vi "DWSPT5_Read.vi"(8 "错误输入（无错误）":errorcluster, 11 "VISA resource name":refnum<visa-resource-name> caption="VISA资源名称") -> (0 "error out":errorcluster caption="错误输出", 3 "Data":T1)   [LabVIEW 2017]
panel:
  out "长度 2":i32
  out "长度":i32
  out "HumidityValue":string
  out "TemperatureValue":string
  in  "Command":string="010300010002\n"
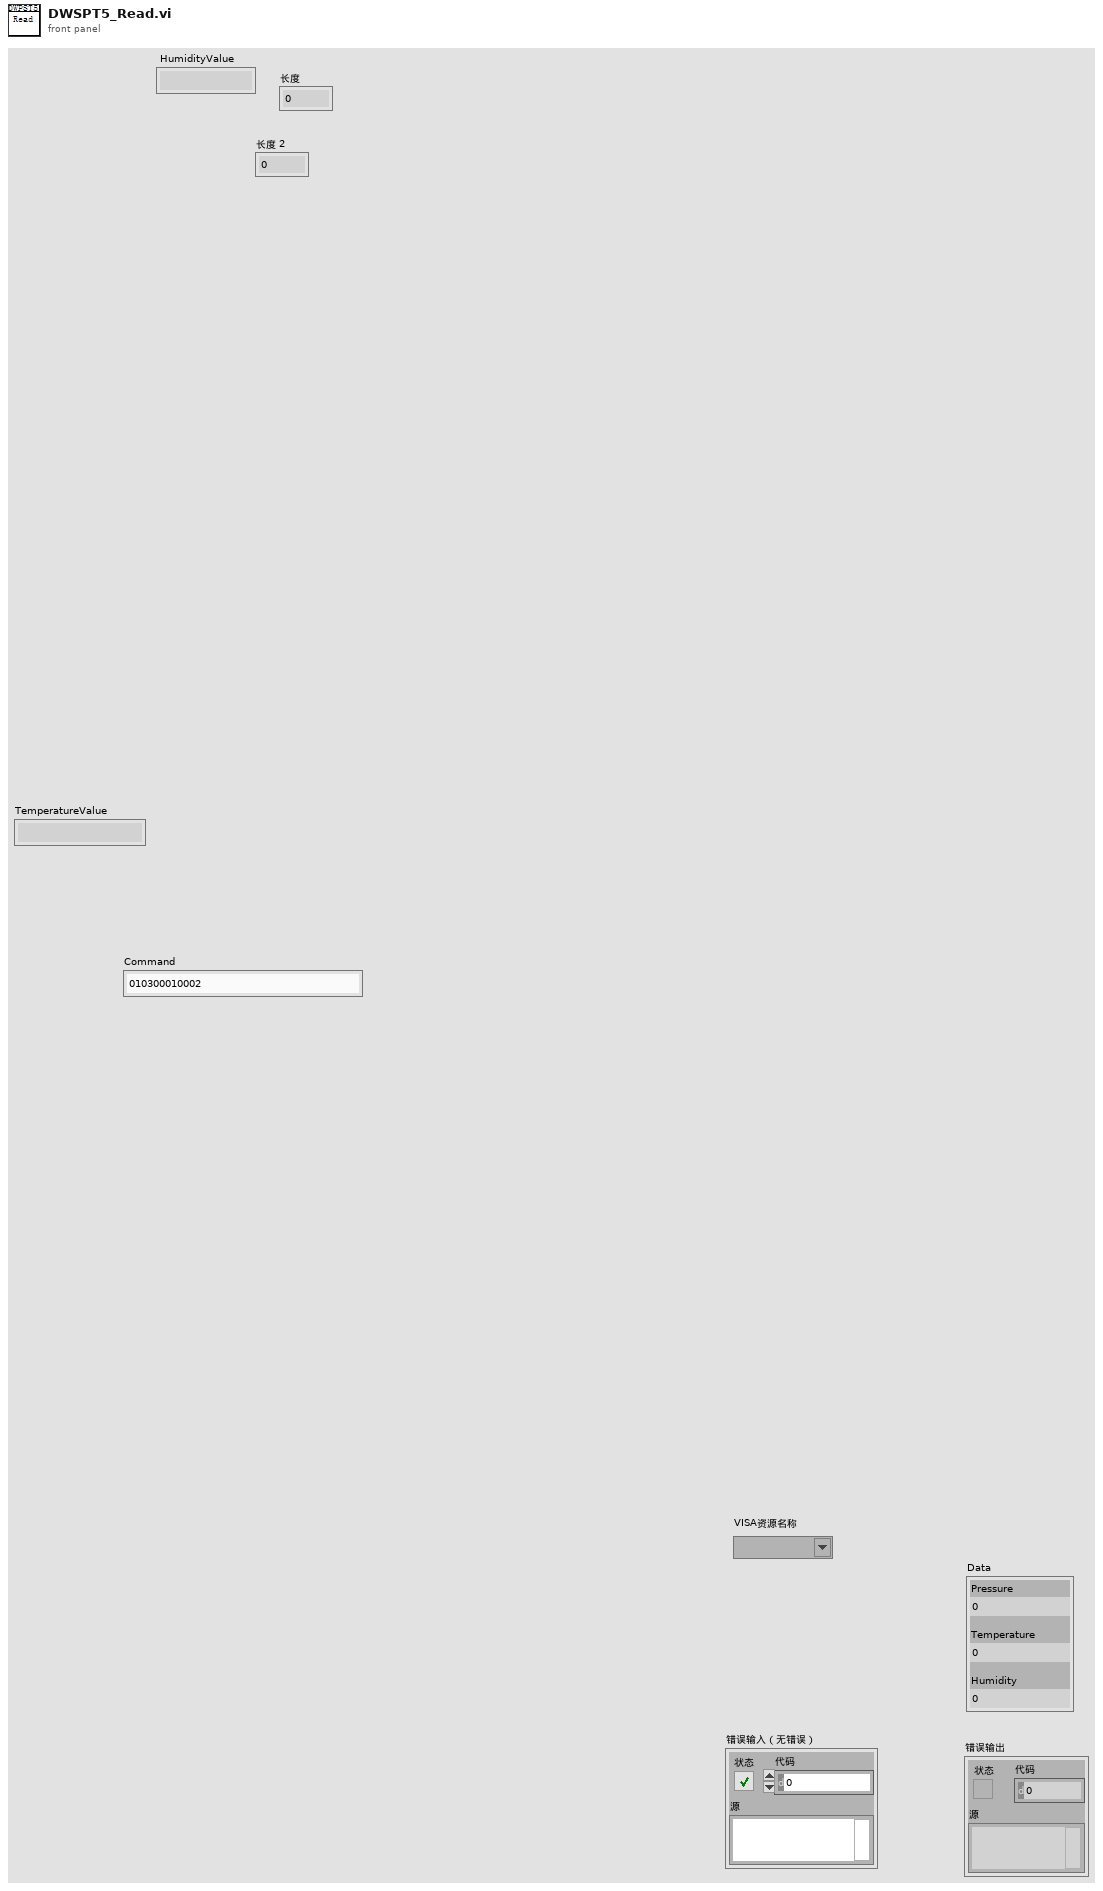
[diagram p1: front panel]
types:
  T1 = cluster{"Pressure":dbl, "Temperature":dbl, "Humidity":dbl}
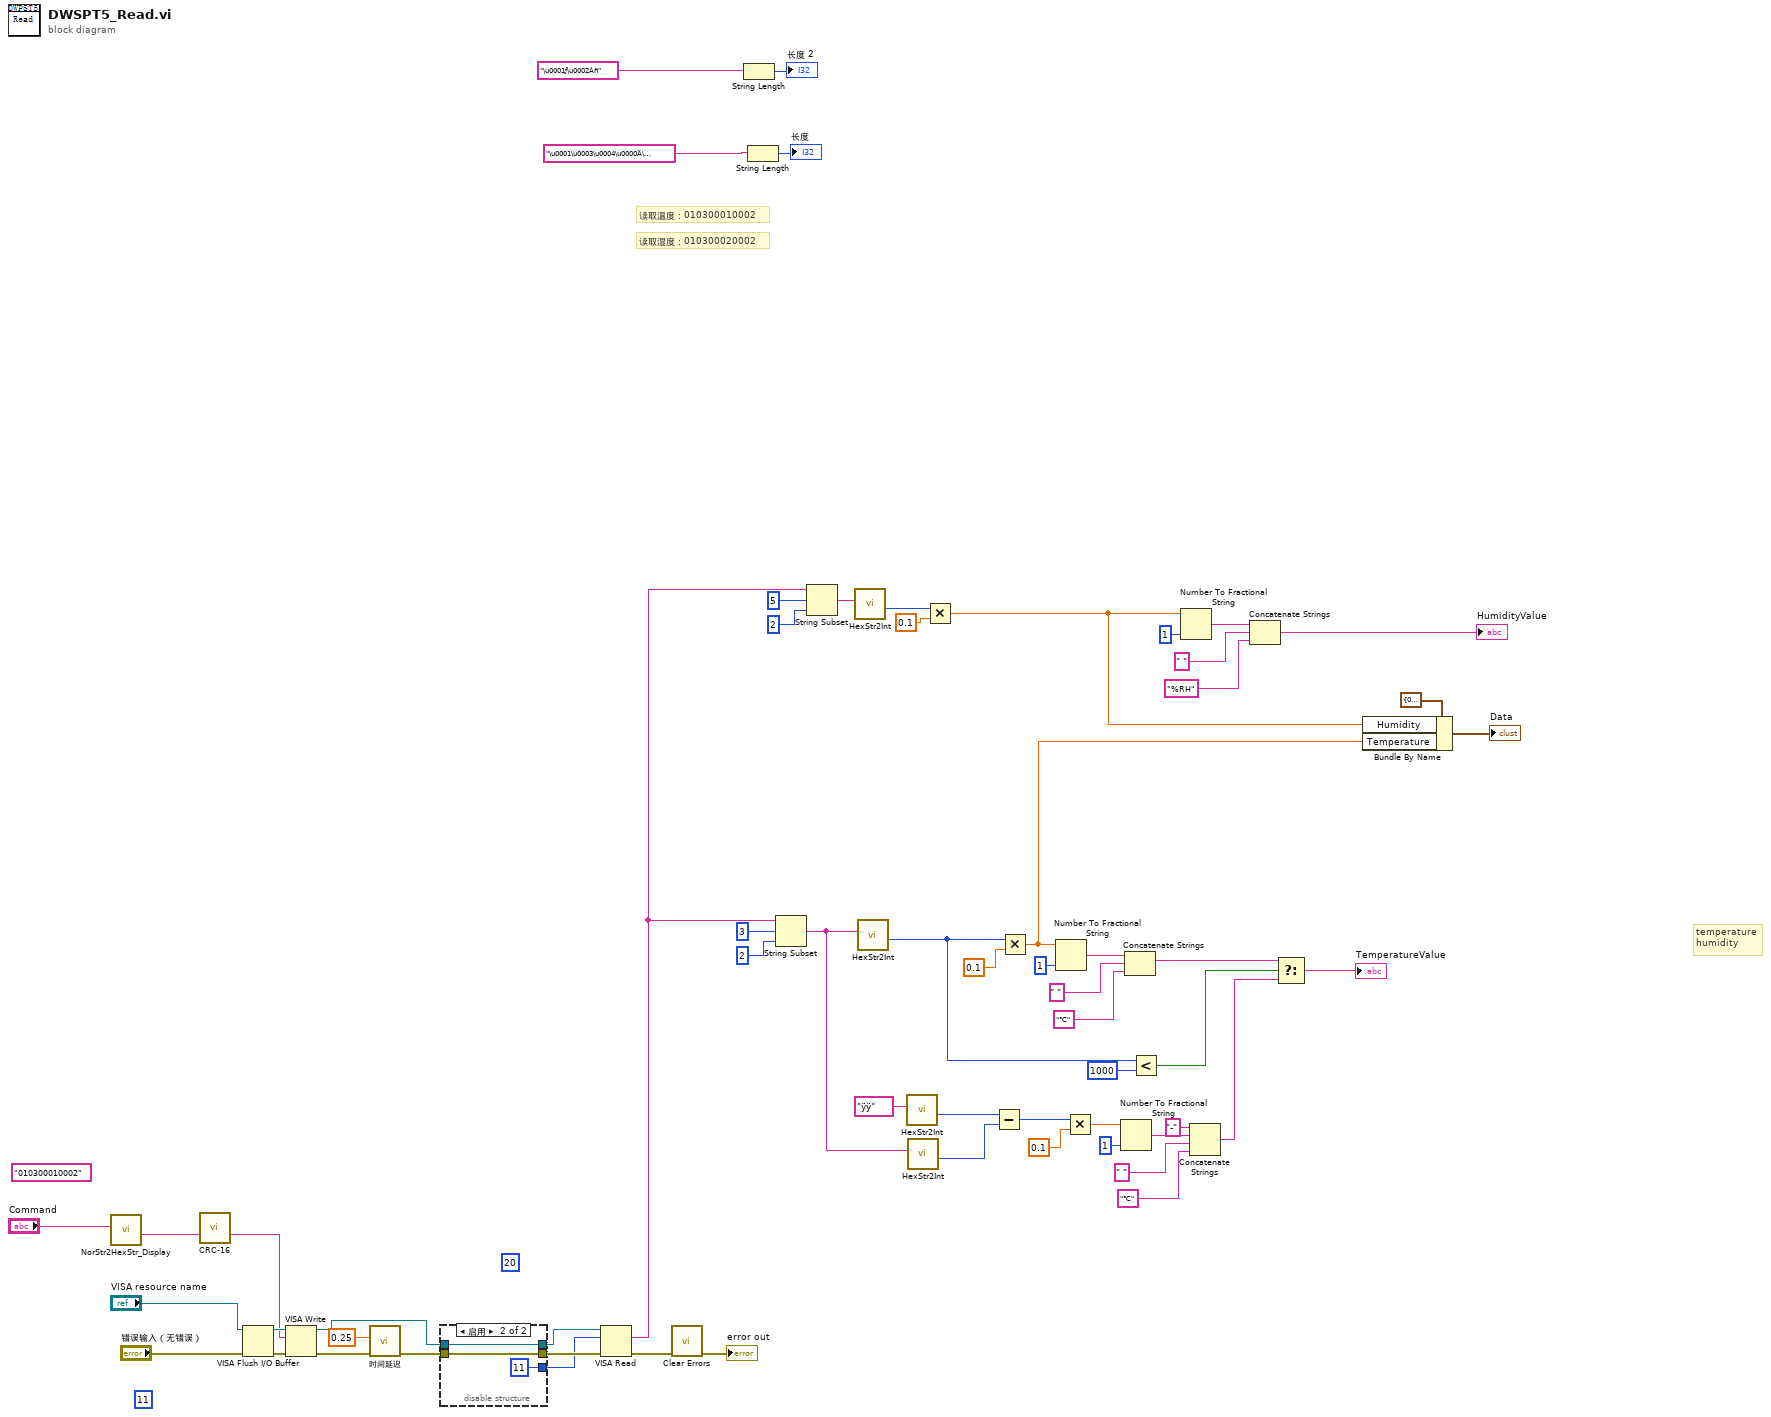
[diagram p0: block diagram]
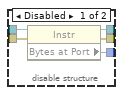
[diagram p2: hidden frame]
diagram:
  (unwired) "010300010002" ("Command 2")
  (unwired) u32 20 ("字节总数")
  (unwired) u32 11 ("byte count")
  # "读取湿度：010300020002"
  # "读取温度：010300010002"
  # "temperature\nhumidity"
  n1 = call "NorStr2HexStr_Display.vi"("Normal Display"="Command") -> ("Hex Display"=w45:string)  [unwired: 10 in]
  n2 = call "CRC-16.vi"("string_hex"=w45) -> ("string&CRC-16"=w44:string)  [unwired: 14 in]
  n3 = VISA Flush I/O Buffer(VISA resource name="VISA resource name", error in (no error)="错误输入（无错误）") -> (VISA resource name out=w60:refnum<visa-resource-name>, error out=w58:errorcluster)  [unwired: 1 in]
  n4 = VISA Write(VISA resource name=w60, write buffer=w44, error in (no error)=w58) -> (VISA resource name out=w50:refnum<visa-resource-name>, error out=w59:errorcluster)  [unwired: 1 out]
  n5 = call "时间延迟"("error in (no error)"=w59, "Delay Time (s)"=0.25) -> ("error out"=w49:errorcluster)  [unwired: 9 in]
  n6 = disable-structure shown="启用" {
    disable-tunnel: w50 -> [w65 w68]
    disable-tunnel: w49 -> [w64 w67]
    disable-tunnel: [w63 w68] -> w48
    disable-tunnel: [w62 w67] -> w47
    disable-tunnel: [w61 u32 11 ("Bytes at Port")] -> w46
    frame Disabled {
      n7 = property class="Instr"(reference=w65, error in=w64) -> (reference out=w63:refnum<visa-resource-name>, error out=w62:errorcluster, "Bytes at Port"=w61:u32)
    }
    frame Enabled {
    }
  }
  n8 = VISA Read(VISA resource name=w48, byte count=w46, error in (no error)=w47) -> (read buffer=w3:string, error out=w57:errorcluster)  [unwired: 2 out]
  n9 = call <vilib>:"Clear Errors.vi"("error in (no error)"=w57) -> ("error out"=→"error out":errorcluster)  [unwired: 5 in, 1 out]
  n10 = String Length(string="\u0001ƒ\u0002Àñ" ("字符串")) -> (length=→"长度 2":i32)
  n11 = String Length(string="\u0001\u0003\u0004\u0000Ä\u00014»‰" ("字符串")) -> (length=→"长度":i32)
  n12 = String Subset(string=w3, offset (0)=3 ("偏移量(0)"), length (rest)=2 ("长度（剩余）")) -> (substring=w19:string)
  n13 = String Subset(string=w3, offset (0)=5 ("偏移量(0)"), length (rest)=2 ("长度（剩余）")) -> (substring=w18:string)
  n14 = call "HexStr2Int.vi"("十六进制字符串"=w18) -> ("数字"=w17:u32)  [unwired: 10 in]
  n15 = call "HexStr2Int.vi"("十六进制字符串"=w19) -> ("数字"=w20:u32)  [unwired: 10 in]
  n16 = call "HexStr2Int.vi"("十六进制字符串"="ÿÿ") -> ("数字"=w34:u32)  [unwired: 10 in]
  n17 = call "HexStr2Int.vi"("十六进制字符串"=w19) -> ("数字"=w33:u32)  [unwired: 10 in]
  n18 = Multiply(x=w17, y=0.1) -> (x*y=w2:dbl)
  n19 = Subtract(x=w34, y=w33) -> (x-y=w26:u32)
  n20 = Multiply(x=w20, y=0.1) -> (x*y=w1:dbl)
  n21 = Number To Fractional String(number=w1, precision (6)=i16 1 ("精度(6)")) -> (F-format string=w36:string)  [unwired: 2 in]
  n22 = Multiply(x=w26, y=0.1) -> (x*y=w28:dbl)
  n23 = Number To Fractional String(number=w28, precision (6)=i16 1 ("精度(6)")) -> (F-format string=w32:string)  [unwired: 2 in]
  n24 = Concatenate Strings(w36, " " ("字符串"), "℃" ("字符串")) -> (w22:string)
  n25 = Less?(x=w20, y=u32 1000) -> (x < y?=w23:bool)
  n26 = Number To Fractional String(number=w2, precision (6)=i16 1 ("精度(6)")) -> (F-format string=w16:string)  [unwired: 2 in]
  n27 = Concatenate Strings("-" ("字符串"), w32, " " ("字符串"), "℃" ("字符串")) -> (w21:string)
  n28 = Concatenate Strings(w16, " " ("字符串"), "%RH" ("字符串")) -> (→"HumidityValue":string)
  n29 = Select(t=w22, s=w23, f=w21) -> (s? t:f=→"TemperatureValue":string)
  n30 = Bundle By Name(cluster=T1 {"Pressure"=0.0, "Temperature"=0.0, "Humidity"=0.0} ("Data"), "Humidity"=w2, "Temperature"=w1) -> (→"Data":T1)
